vi "Clear.vi"(8 "error in (no error)":errorcluster, 11 "View In":refnum<class "View.lvclass">) -> (0 "error out":errorcluster)   [LabVIEW 2020, in "View.lvclass"]
doc: "Clears any resorces allocated during initialization."
uses:
  View.lvclass
  View.lvclass/View.ctl
  Process/Process.lvclass
  C:/git/astemes-triarc-framework/source/Framework/Process/Process.lvclass
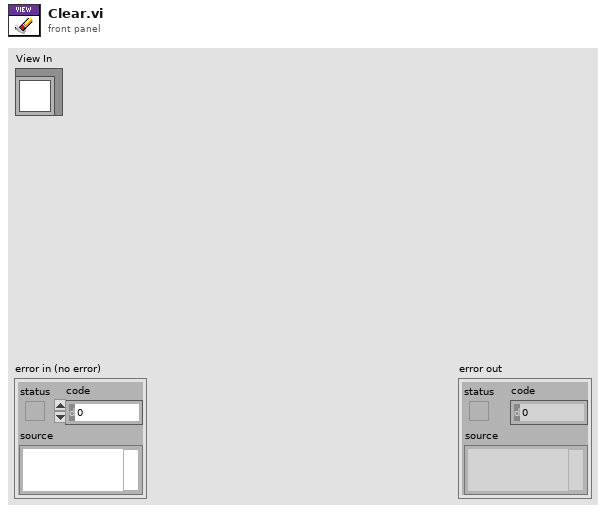
[diagram p1: front panel]
types:
  T1 = typedef "Process.lvclass/Lifecycle State.ctl" = enum16{"Uninitialized", "Initialized", "Started", "Running", "Stopped", "Finished"}
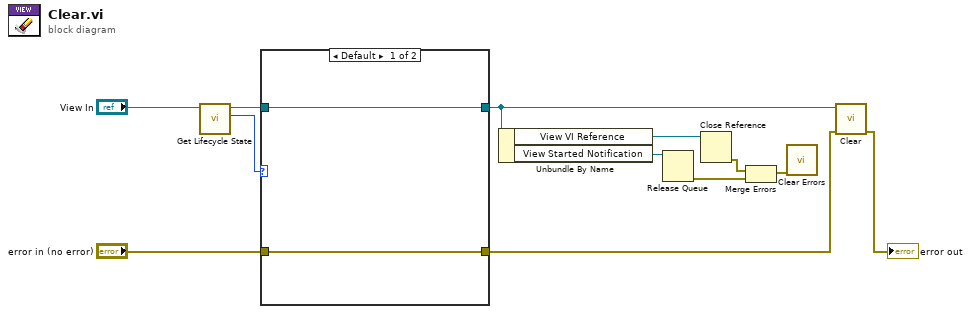
[diagram p0: block diagram]
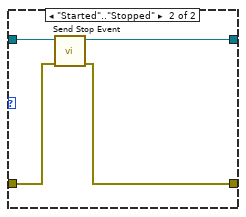
[diagram p2: hidden frame]
diagram:
  n1 = call "Get Lifecycle State.vi"("Process In"="View In") -> ("Lifecycle State"=w10:T1, "Process Out"=w11:refnum<class "View.lvclass">)  [unwired: 7 in, 2 out]
  n2 = case shown="Default" w10 {
    tunnel: [w13 w17] -> w8
    tunnel: w11 -> [w14 w16]
    tunnel: "error in (no error)" -> [w13 w18]
    tunnel: [w14 w15] -> w5
    frame Default {
    }
    frame "Started".."Stopped" {
      n3 = call "Send Stop Event.vi"("error in (no error)"=w18, "View In"=w16) -> ("error out"=w17:errorcluster, "View Out"=w15:refnum<class "View.lvclass">)  [unwired: 8 in]
    }
  }
  n4 = Unbundle By Name(w5) -> ("View VI Reference"=w4:refnum<vi>, "View Started Notification"=w6:refnum<queue>)
  n5 = Release Queue(queue=w6) -> (error out=w2:errorcluster)  [unwired: 2 in, 2 out]
  n6 = Close Reference(reference=w4) -> (error out=w3:errorcluster)  [unwired: 1 in]
  n7 = Merge Errors(w3, w2) -> (w1:errorcluster)
  n8 = call <vilib>:"Clear Errors.vi"("error in (no error)"=w1) -> ()  [unwired: 5 in, 2 out]
  n9 = call-parent "Clear.vi"("error in (no error)"=w8, "Process In"=w5) -> ("error out"=→"error out":errorcluster)  [unwired: 9 in]
